vi "baseUrl.get.vi"(11 "series_class in":refnum<class "series_class.lvclass">) -> (2 "base url":string, 3 "series_class out":refnum<class "series_class.lvclass">)   [LabVIEW 2024, in "series_class.lvclass"]
uses:
  series_class.lvclass
  series_class.lvclass/series_class.ctl
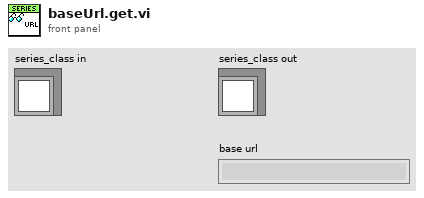
[diagram p1: front panel]
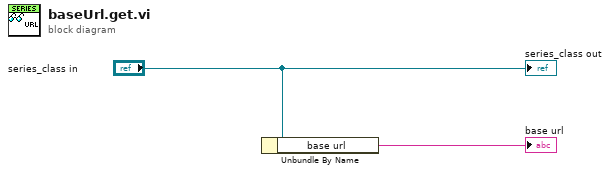
[diagram p0: block diagram]
diagram:
  n1 = Unbundle By Name("series_class in") -> ("base url"=→"base url":string)
  "series_class out" <- "series_class in"
